vi "Excel Files.vi"   [LabVIEW 2013]
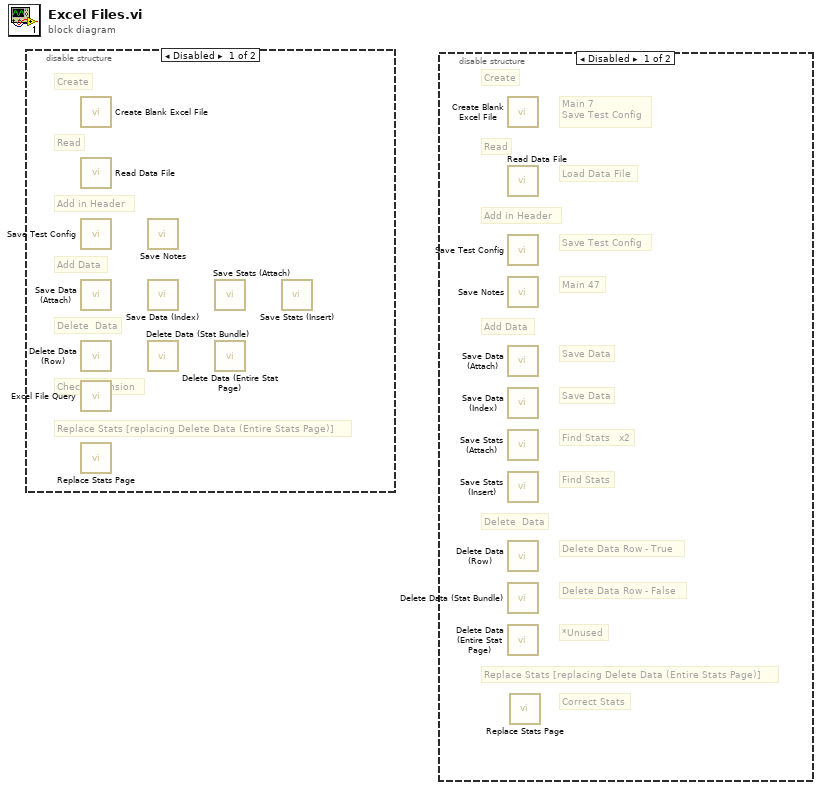
[diagram p0: block diagram]
diagram:
  n1 = disable-structure shown="Disabled" {
    frame Disabled {
      # "Replace Stats [replacing Delete Data (Entire Stats Page)]"
      # "Check Extension"
      # "Delete  Data"
      # "Add Data"
      # "Add in Header"
      # "Read"
      # "Create"
      n2 = call "Create Blank Excel File.vi"() -> ()  [unwired: 13 in, 3 out]
      n3 = call "Read Data File.vi"() -> ()  [unwired: 5 in, 11 out]
      n4 = call "Save Test Config.vi"() -> ()  [unwired: 15 in, 1 out]
      n5 = call "Save Data (Attach).vi"() -> ()  [unwired: 15 in, 1 out]
      n6 = call "Delete Data (Row).vi"() -> ()  [unwired: 15 in, 1 out]
      n7 = call "Excel File Query.vi"() -> ()  [unwired: 5 in, 1 out]
      n8 = call "Replace Stats Page.vi"() -> ()  [unwired: 15 in, 1 out]
      n9 = call "Save Notes.vi"() -> ()  [unwired: 15 in, 1 out]
      n10 = call "Save Data (Index).vi"() -> ()  [unwired: 15 in, 1 out]
      n11 = call "Delete Data (Stat Bundle).vi"() -> ()  [unwired: 15 in, 1 out]
      n12 = call "Save Stats (Attach).vi"() -> ()  [unwired: 15 in, 1 out]
      n13 = call "Delete Data (Entire Stat Page).vi"() -> ()  [unwired: 15 in, 1 out]
      n14 = call "Save Stats (Insert).vi"() -> ()  [unwired: 15 in, 1 out]
    }
    frame Enabled {
    }
  }
  n15 = disable-structure shown="Disabled" {
    frame Disabled {
      # "Correct Stats"
      # "Replace Stats [replacing Delete Data (Entire Stats Page)]"
      # "*Unused"
      # "Delete Data Row - False"
      # "Delete Data Row - True"
      # "Find Stats"
      # "Find Stats   x2"
      # "Save Data"
      # "Save Data"
      # "Main 47"
      # "Save Test Config"
      # "Load Data File"
      # "Main 7\nSave Test Config"
      # "Delete  Data"
      # "Add Data"
      # "Add in Header"
      # "Read"
      # "Create"
      n16 = call "Create Blank Excel File.vi"() -> ()  [unwired: 13 in, 3 out]
      n17 = call "Read Data File.vi"() -> ()  [unwired: 5 in, 11 out]
      n18 = call "Save Test Config.vi"() -> ()  [unwired: 15 in, 1 out]
      n19 = call "Save Notes.vi"() -> ()  [unwired: 15 in, 1 out]
      n20 = call "Save Data (Attach).vi"() -> ()  [unwired: 15 in, 1 out]
      n21 = call "Save Data (Index).vi"() -> ()  [unwired: 15 in, 1 out]
      n22 = call "Save Stats (Attach).vi"() -> ()  [unwired: 15 in, 1 out]
      n23 = call "Save Stats (Insert).vi"() -> ()  [unwired: 15 in, 1 out]
      n24 = call "Delete Data (Row).vi"() -> ()  [unwired: 15 in, 1 out]
      n25 = call "Delete Data (Stat Bundle).vi"() -> ()  [unwired: 15 in, 1 out]
      n26 = call "Delete Data (Entire Stat Page).vi"() -> ()  [unwired: 15 in, 1 out]
      n27 = call "Replace Stats Page.vi"() -> ()  [unwired: 15 in, 1 out]
    }
    frame Enabled {
    }
  }
